vi "Start Tasks.vi"(8 "error in":errorcluster, 10 "Red Tasks":T1={"CLk"="CRDS Red Clk", "AI"="CRDS Red AI", "DO"="CRD Red Laser Output"}, 11 "Blue Tasks":T1={"CLk"="CRDS Red Clk", "AI"="CRDS Red AI", "DO"="CRD Red Laser Output"}) -> (0 "error out":errorcluster)   [LabVIEW 2014, in "eCRDS Library.lvlib" / "Update Laser rate and DC.lvclass"]
uses:
  Update Laser rate and DC.lvclass
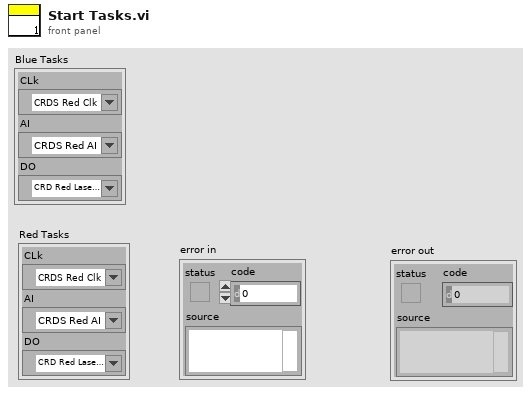
[diagram p1: front panel]
types:
  T1 = cluster{"CLk":refnum<k21>, "AI":refnum<k21>, "DO":refnum<k21>}
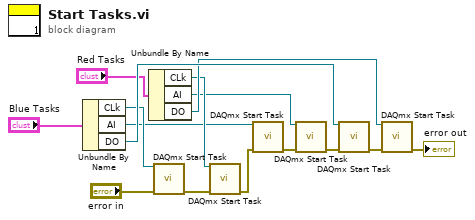
[diagram p0: block diagram]
diagram:
  n1 = Unbundle By Name("Blue Tasks") -> ("CLk"=w9:refnum<k21>, "AI"=w5:refnum<k21>, "DO"=w14:refnum<k21>)
  n2 = Unbundle By Name("Red Tasks") -> ("CLk"=w7:refnum<k21>, "AI"=w4:refnum<k21>, "DO"=w12:refnum<k21>)
  n3 = call <vilib>:"DAQmx Start Task.vi"("task/channels in"=w9, "error in"="error in") -> ("error out"=w6:errorcluster)  [unwired: 12 in, 1 out]
  n4 = call <vilib>:"DAQmx Start Task.vi"("task/channels in"=w7, "error in"=w6) -> ("error out"=w3:errorcluster)  [unwired: 12 in, 1 out]
  n5 = call <vilib>:"DAQmx Start Task.vi"("task/channels in"=w5, "error in"=w3) -> ("error out"=w2:errorcluster)  [unwired: 12 in, 1 out]
  n6 = call <vilib>:"DAQmx Start Task.vi"("task/channels in"=w4, "error in"=w2) -> ("error out"=w1:errorcluster)  [unwired: 12 in, 1 out]
  n7 = call <vilib>:"DAQmx Start Task.vi"("task/channels in"=w14, "error in"=w1) -> ("error out"=w11:errorcluster)  [unwired: 12 in, 1 out]
  n8 = call <vilib>:"DAQmx Start Task.vi"("task/channels in"=w12, "error in"=w11) -> ("error out"=→"error out":errorcluster)  [unwired: 12 in, 1 out]
